vi "Ref_Num_Stopwatch_Sh.vi"(0 "Elapsed time (seconds)":refnum<vi>, 2 "start time":refnum<vi>, 3 "Started":refnum<vi>, 4 "OK Button":refnum<vi>, 5 "stop":refnum<vi>) -> ()   [LabVIEW 2020]
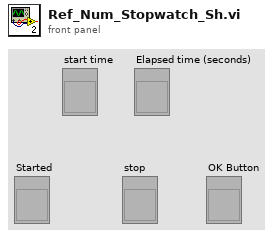
[diagram p1: front panel]
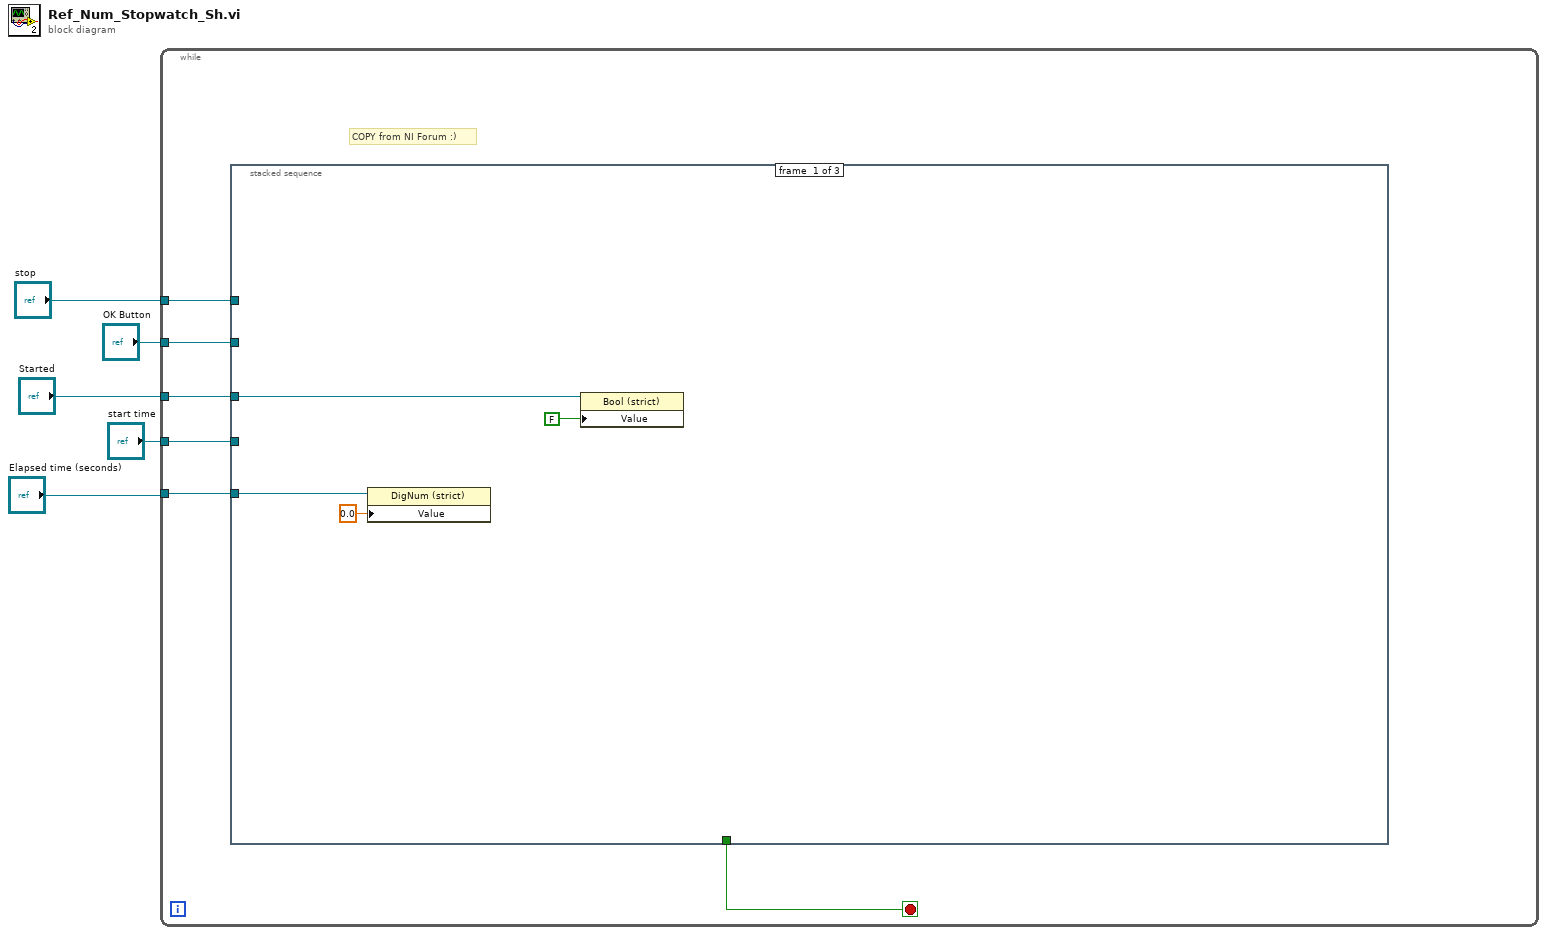
[diagram p0: block diagram]
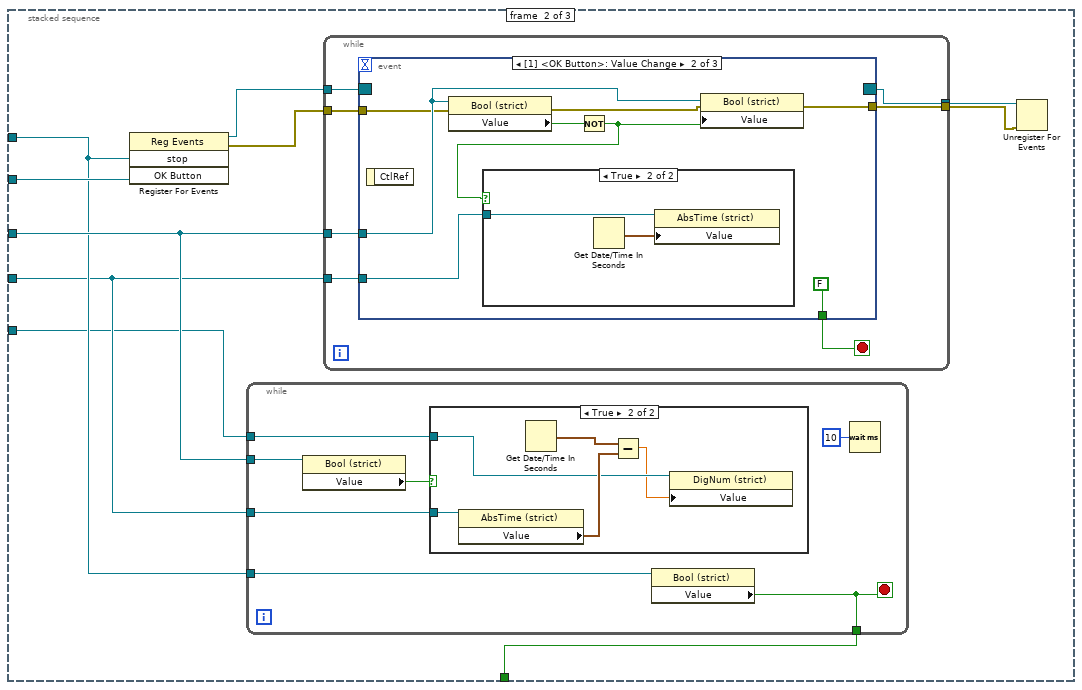
[diagram p2: hidden frame]
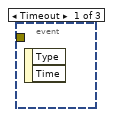
[diagram p4: hidden frame]
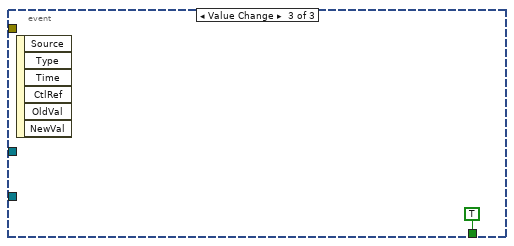
[diagram p6: hidden frame]
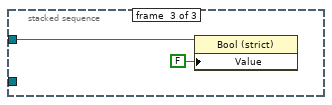
[diagram p7: hidden frame]
diagram:
  n1 = while {
    tunnel: "Started" -> [w11]
    tunnel: "OK Button" -> [w10]
    tunnel: "Elapsed time (seconds)" -> [w9]
    tunnel: "stop" -> [w8]
    tunnel: "start time" -> [w7]
    stop <- w6 stop-if-true
    # "COPY from NI Forum :)"
    n2 = stacked-sequence {
      tunnel: [_ w25 _] -> w6
      tunnel: w11 -> [w15 w22 _]
      tunnel: w10 -> [_ w24 _]
      tunnel: w9 -> [w13 w19 _]
      tunnel: w8 -> [_ w21 w57]
      tunnel: w7 -> [_ w20 _]
      frame #0 {
        n3 = property class="DigNum (strict)"(reference=w13, "Value"=0.0 ("Elapsed time (seconds)")) -> ()  [unwired: 1 in, 2 out]
        n4 = property class="Bool (strict)"(reference=w15, "Value"=FALSE ("Started")) -> ()  [unwired: 1 in, 2 out]
      }
      frame #1 {
        n5 = register-events(w21, w24) -> (reference out=w23:refnum<event-registration>, error out=w17:errorcluster)  [unwired: 2 in]
        n6 = while {
          tunnel: [w28] -> w25
          tunnel: w22 -> [w31]
          tunnel: w21 -> [w29]
          tunnel: w20 -> [w27]
          tunnel: w19 -> [w26]
          stop <- w28 stop-if-true
          n7 = property class="Bool (strict)"(reference=w31) -> ("Value"=w30:bool)  [unwired: 1 in, 2 out]
          n8 = case shown="True" w30 {
            tunnel: w27 -> [_ w36]
            tunnel: w26 -> [_ w34]
            frame False {
              # "do nothing"
            }
            frame True {
              n9 = property class="AbsTime (strict)"(reference=w36) -> ("Value"=w35:timestamp)  [unwired: 1 in, 2 out]
              n10 = Get Date/Time In Seconds() -> (seconds since 1Jan1904=w37:timestamp)
              n11 = Subtract(x=w37, y=w35) -> (x-y=w33:dbl)
              n12 = property class="DigNum (strict)"(reference=w34, "Value"=w33) -> ()  [unwired: 1 in, 2 out]
            }
          }
          n13 = property class="Bool (strict)"(reference=w29) -> ("Value"=w28:bool)  [unwired: 1 in, 2 out]
          n14 = Wait (ms)(milliseconds to wait=u32 10) -> ()  [unwired: 1 out]
        }
        n15 = while {
          tunnel: w23 -> [w43]
          tunnel: w22 -> [w42]
          tunnel: w20 -> [w41]
          tunnel: [w40] -> w18
          tunnel: w17 -> [w39]
          tunnel: [w38] -> w16
          stop <- w44 stop-if-true
          n16 = event shown="[1] <OK Button>: Value Change" {
            selector: w43 -> [_ _ _]
            dyn-events: [_ _ _] -> w40
            timeout: _ -> [_ _ _]
            tunnel: [_ FALSE TRUE] -> w44
            tunnel: w42 -> [_ w51 _]
            tunnel: w41 -> [_ w48 _]
            tunnel: w39 -> [_ w47 _]
            tunnel: [_ w45 _] -> w38
            event Timeout {
              n17 = event-data() -> ()  [unwired: 1 in, 2 out]
            }
            event Value Change {
              n18 = event-data() -> ()  [unwired: 1 in, 1 out]
              n19 = property class="Bool (strict)"(reference=w51, error in=w47) -> (error out=w46:errorcluster, "Value"=w50:bool)  [unwired: 1 out]
              n20 = Not(x=w50) -> (.not. x?=w49:bool)
              n21 = case shown="True" w49 {
                tunnel: w48 -> [_ w54]
                frame False {
                }
                frame True {
                  n22 = Get Date/Time In Seconds() -> (seconds since 1Jan1904=w53:timestamp)
                  n23 = property class="AbsTime (strict)"(reference=w54, "Value"=w53) -> ()  [unwired: 1 in, 2 out]
                }
              }
              n24 = property class="Bool (strict)"(reference=w51, error in=w46, "Value"=w49) -> (error out=w45:errorcluster)  [unwired: 1 out]
            }
            event Value Change {
              n25 = event-data() -> ()  [unwired: 1 in, 6 out]
            }
          }
        }
        n26 = Unregister For Events(event registration refnum=w18, error in=w16) -> ()  [unwired: 1 out]
      }
      frame #2 {
        n27 = property class="Bool (strict)"(reference=w57, "Value"=FALSE) -> ()  [unwired: 1 in, 2 out]
      }
    }
  }
